vi "closed drive.vi"(2 "Y axis value":dbl, 3 "X axis value":dbl) -> (0 "right":dbl format="%.2f", 1 "left":dbl format="%.2f")   [LabVIEW 2011]
doc: "Holds the drivetrain position, so the robot resists movement. This is useful when balancing bridges. It's like a software brake... This VI also allows for the driver to make slight adjustments in robot position."
uses:
  <vilib>/addons/control/pid/pid.llb/PID (DBL).vi
  <vilib>/addons/control/pid/NI_PID_pid.lvlib
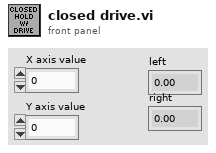
[diagram p1: front panel]
types:
  T1 = typedef "WPI_EncoderDevRef.ctl" = cluster{"DevStatus":errorcluster, "EncoderIndex":T2, "CounterIndex":T3, "DistancePerCount":dbl, "Decoding Type":T4}
  T2 = typedef "FPGA_EncoderIdx.ctl" = enum8{"Enc 0", "Enc 1", "Enc 2", "Enc 3", "Invalid"}
  T3 = typedef "FPGA_CounterCtrSystemIndex.ctl" = enum8{"Ctr 0", "Ctr 1", "Ctr 2", "Ctr 3", "Ctr 4", "Ctr 5", "Ctr 6", "Ctr 7", "Invalid"}
  T4 = typedef "WPI_EncoderType.ctl" = enum16{"1x", "2x", "4x"}
  T5 = cluster{"proportional gain (Kc)":dbl, "integral time (Ti, min)":dbl, "derivative time (Td, min)":dbl}
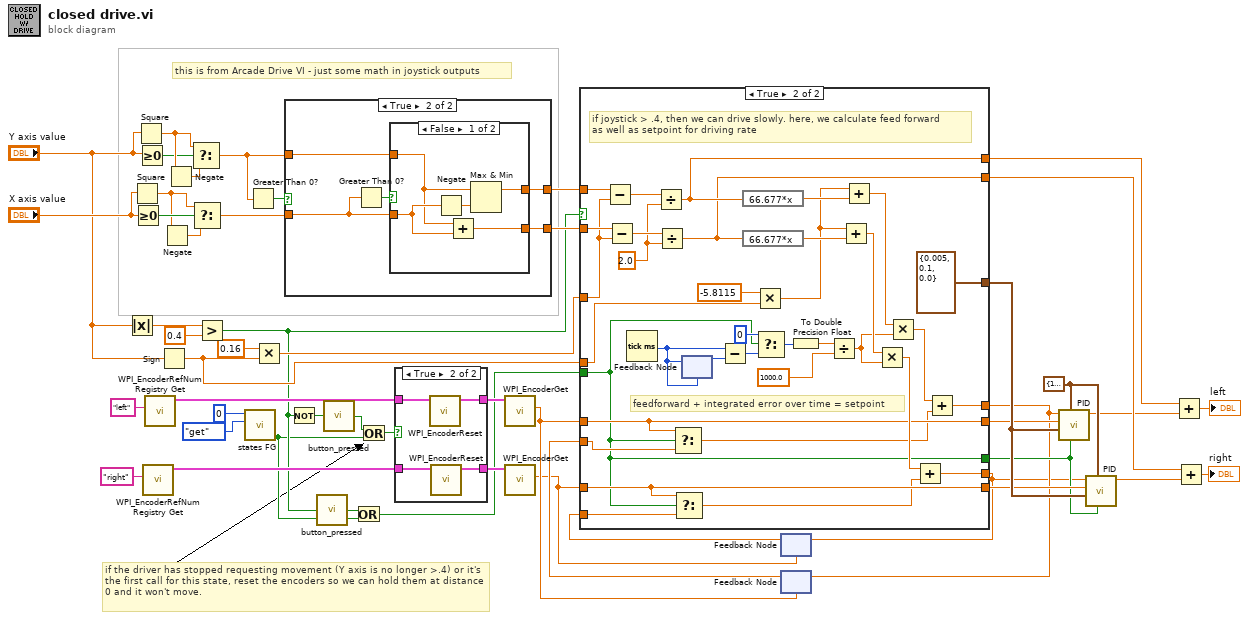
[diagram p0: block diagram]
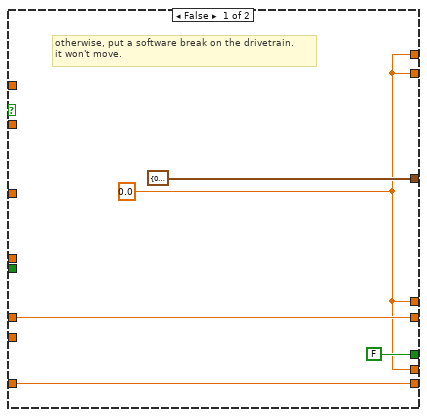
[diagram p2: hidden frame]
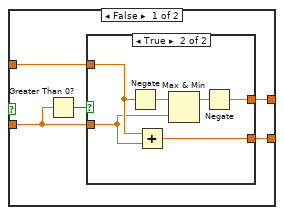
[diagram p3: hidden frame]
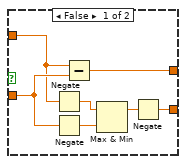
[diagram p4: hidden frame]
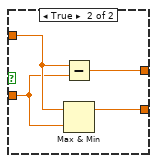
[diagram p5: hidden frame]
diagram:
  w46 = cluster{"output high":dbl, "output low":dbl} {"output high"=1.0, "output low"=-1.0} ("output range")
  # "if the driver has stopped requesting movement (Y axis is no longer >.4) or it's the first call for this state, reset the encoders so we can hold them at distance 0 and it won't move."
  # "this is from Arcade Drive VI - just some math in joystick outputs"
  n1 = Absolute Value(x="Y axis value") -> (abs(x)=w25:dbl)
  n2 = Square(x="X axis value") -> (x^2=w36:dbl)
  n3 = Greater Or Equal To 0?(x="X axis value") -> (x >= 0?=w37:bool)
  n4 = Square(x="Y axis value") -> (x^2=w33:dbl)
  n5 = Greater Or Equal To 0?(x="Y axis value") -> (x >= 0?=w32:bool)
  n6 = call <vilib>:"WPI_EncoderRefNum Registry Get.vi"("refnum name"="right") -> ("EncoderDevRef"=w47:T1)  [unwired: 9 in, 1 out]
  n7 = call <vilib>:"WPI_EncoderRefNum Registry Get.vi"("refnum name"="left") -> ("EncoderDevRef"=w48:T1)  [unwired: 9 in, 1 out]
  n8 = Sign(1:"Y axis value") -> (0:w16:dbl)
  n9 = Negate(x=w36) -> (-x=w35:dbl)
  n10 = Negate(x=w33) -> (-x=w34:dbl)
  n11 = Select(t=w33, s=w32, f=w34) -> (s? t:f=w40:dbl)
  n12 = Select(t=w36, s=w37, f=w35) -> (s? t:f=w39:dbl)
  n13 = Greater?(x=w25, y=0.4) -> (0:w2:bool)
  n14 = call "states FG.vi"("menu (get)"=enum16{"set", "get"}."get", "Loop ID"=0) -> ("first call?"=w1:bool)  [unwired: 6 in, 3 out]
  n15 = Greater Than 0?(x=w40) -> (x > 0?=w41:bool)
  n16 = Multiply(x=0.16, y=w16) -> (x*y=w17:dbl)
  n17 = case shown="True" w41 {
    tunnel: w39 -> [w54 w72]
    tunnel: w40 -> [w53 w71]
    tunnel: [w52 w70] -> w31
    tunnel: [w51 w69] -> w30
    frame False {
      n18 = Greater Than 0?(x=w54) -> (x > 0?=w55:bool)
      n19 = case shown="True" w55 {
        tunnel: w54 -> [w62 w64]
        tunnel: w53 -> [w60 w65]
        tunnel: [w56 w66] -> w52
        tunnel: [w57 w63] -> w51
        frame False {
          n20 = Negate(x=w60) -> (-x=w61:dbl)
          n21 = Negate(x=w62) -> (-x=w59:dbl)
          n22 = Subtract(x=w60, y=w62) -> (x-y=w56:dbl)
          n23 = Max & Min(x=w61, y=w59) -> (max(x,y)=w58:dbl)  [unwired: 1 out]
          n24 = Negate(x=w58) -> (-x=w57:dbl)
        }
        frame True {
          n25 = Negate(x=w65) -> (-x=w68:dbl)
          n26 = Add(x=w65, y=w64) -> (x+y=w63:dbl)
          n27 = Max & Min(x=w68, y=w64) -> (max(x,y)=w67:dbl)  [unwired: 1 out]
          n28 = Negate(x=w67) -> (-x=w66:dbl)
        }
      }
    }
    frame True {
      n29 = Greater Than 0?(x=w72) -> (x > 0?=w73:bool)
      n30 = case shown="False" w73 {
        tunnel: w72 -> [w78 w80]
        tunnel: w71 -> [w75 w81]
        tunnel: [w76 w79] -> w70
        tunnel: [w74 w82] -> w69
        frame False {
          n31 = Negate(x=w78) -> (-x=w77:dbl)
          n32 = Add(x=w75, y=w78) -> (x+y=w74:dbl)
          n33 = Max & Min(x=w75, y=w77) -> (max(x,y)=w76:dbl)  [unwired: 1 out]
        }
        frame True {
          n34 = Subtract(x=w81, y=w80) -> (x-y=w79:dbl)
          n35 = Max & Min(x=w81, y=w80) -> (max(x,y)=w82:dbl)  [unwired: 1 out]
        }
      }
    }
  }
  n36 = Not(x=w2) -> (.not. x?=w19:bool)
  n37 = call "button_pressed.vi"("Button In"=w2) -> ("Button Pressed?"=w4:bool)
  n38 = call "button_pressed.vi"("Button In"=w19) -> ("Button Pressed?"=w22:bool)
  n39 = Or(x=w4, y=w1) -> (x .or. y?=w3:bool)
  n40 = Or(x=w22, y=w1) -> (x .or. y?=w23:bool)
  n41 = case shown="True" w23 {
    tunnel: w48 -> [w84 w88]
    tunnel: w47 -> [w83 w87]
    tunnel: [w84 w86] -> w45
    tunnel: [w83 w85] -> w44
    frame False {
    }
    frame True {
      n42 = call <vilib>:"WPI_EncoderReset.vi"("EncoderDevRef"=w88) -> ("EncoderDevRef"=w86:T1)  [unwired: 9 in, 1 out]
      n43 = call <vilib>:"WPI_EncoderReset.vi"("EncoderDevRef"=w87) -> ("EncoderDevRef"=w85:T1)  [unwired: 9 in, 1 out]
    }
  }
  n44 = call <vilib>:"WPI_EncoderGet.vi"("EncoderDevRef"=w45) -> ("Distance"=w6:dbl)  [unwired: 5 in, 5 out]
  n45 = call <vilib>:"WPI_EncoderGet.vi"("EncoderDevRef"=w44) -> ("Distance"=w5:dbl)  [unwired: 5 in, 5 out]
  n46 = feedback #1(w5) -> (w8:dbl)
  n47 = feedback #2(w6) -> (w10:dbl)
  n48 = case shown="True" w2 {
    tunnel: w31 -> [_ w128]
    tunnel: w30 -> [_ w127]
    tunnel: w17 -> [_ w126]
    tunnel: [w89 w103] -> w9
    tunnel: [w89 w102] -> w7
    tunnel: [T5 {"proportional gain (Kc)"=0.08, "integral time (Ti, min)"=0.0, "derivative time (Td, min)"=0.0} ("PID gains") T5 {"proportional gain (Kc)"=0.005, "integral time (Ti, min)"=0.1, "derivative time (Td, min)"=0.0} ("PID gains")] -> w28
    tunnel: [w92 w99] -> w21
    tunnel: [w91 w96] -> w20
    tunnel: w6 -> [w92 w99]
    tunnel: w5 -> [w91 w96]
    tunnel: w16 -> [_ w118]
    tunnel: [w89 w116] -> w15
    tunnel: [w89 w115] -> w14
    tunnel: [FALSE ("Button Pressed?") w94] -> w11
    tunnel: w10 -> [_ w100]
    tunnel: w8 -> [_ w97]
    tunnel: w3 -> [_ w94]
    frame False {
      w89 = 0.0
      # "otherwise, put a software break on the drivetrain. \nit won't move."
    }
    frame True {
      w123 = 2.0 ("y")
      # "feedforward + integrated error over time = setpoint"
      # "if joystick > .4, then we can drive slowly. here, we calculate feed forward\nas well as setpoint for driving rate"
      n49 = Subtract(x=w128, y=w126) -> (x-y=w125:dbl)
      n50 = Subtract(x=w127, y=w126) -> (x-y=w124:dbl)
      n51 = Tick Count (ms)() -> (millisecond timer value=w113:u32)
      n52 = Divide(x=w125, y=w123) -> (x/y=w116:dbl)
      n53 = Divide(x=w124, y=w123) -> (x/y=w115:dbl)
      n54 = Select(t=w99, s=w94, f=w100) -> (s? t:f=w98:dbl)
      n55 = Select(t=w96, s=w94, f=w97) -> (s? t:f=w95:dbl)
      n56 = feedback-in #3(w113) -> ()
      n57 = feedback #3(w113) -> (w114:u32)
      n58 = Subtract(x=w113, y=w114) -> (x-y=w112:u32)
      n59 = expression code="66.677*x"(w116) -> (w122:dbl)
      n60 = expression code="66.677*x"(w115) -> (w121:dbl)
      n61 = Multiply(x=-5.8115 ("y"), y=w118) -> (x*y=w117:dbl)
      n62 = Select(t=u32 0, s=w94, f=w112) -> (s? t:f=w110:u32)
      n63 = To Double Precision Float(number=w110) -> (double precision float=w101:dbl)
      n64 = Divide(x=w101, y=1000.0) -> (x/y=w106:dbl)
      n65 = Add(x=w117, y=w121) -> (x+y=w107:dbl)
      n66 = Add(x=w117, y=w122) -> (x+y=w108:dbl)
      n67 = Multiply(x=w107, y=w106) -> (x*y=w104:dbl)
      n68 = Multiply(x=w108, y=w106) -> (x*y=w105:dbl)
      n69 = Add(x=w104, y=w95) -> (x+y=w102:dbl)
      n70 = Add(x=w105, y=w98) -> (x+y=w103:dbl)
    }
  }
  n71 = feedback-in #1(w7) -> ()
  n72 = feedback-in #2(w9) -> ()
  n73 = call-poly <vilib>:"PID.vi"("reinitialize? (F)"=w11, "output range"=w46, "PID gains"=w28, "process variable"=w21, "setpoint"=w9) -> ("output"=w13:dbl)  [unwired: 5 in, 1 out]
  n74 = call-poly <vilib>:"PID.vi"("reinitialize? (F)"=w11, "output range"=w46, "PID gains"=w28, "process variable"=w20, "setpoint"=w7) -> ("output"=w12:dbl)  [unwired: 5 in, 1 out]
  n75 = Add(x=w15, y=w13) -> (x+y=→"left":dbl)
  n76 = Add(x=w14, y=w12) -> (x+y=→"right":dbl)
